vi "Lacie_20_Convertion.vi"(1 "Path":path) -> (0 "Path 2":path)   [LabVIEW 2010]
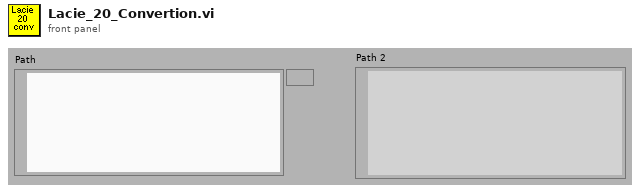
[diagram p1: front panel]
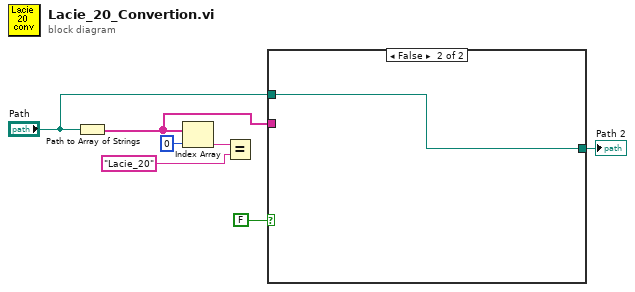
[diagram p0: block diagram]
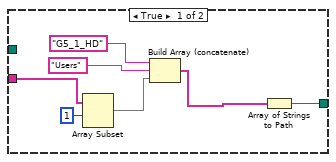
[diagram p2: hidden frame]
diagram:
  n1 = Path to Array of Strings(0:"Path") -> (2:w2:string[])  [unwired: 1 out]
  n2 = Index Array(array=w2, index=0) -> (element=w4:string)
  n3 = Equal?(x=w4, y="Lacie_20" ("regular expression")) -> ()  [unwired: 1 out]
  n4 = case shown="False" FALSE {
    tunnel: [w8 w15] -> w7
    tunnel: "Path" -> [_ w15]
    tunnel: w2 -> [w12 _]
    frame True {
      n5 = Array Subset(array=w12, index=1) -> (w10:string[])  [unwired: 1 in]
      n6 = Build Array (concatenate)("G5_1_HD", "Users", w10) -> (w9:string[])
      n7 = Array of Strings to Path(0:w9) -> (2:w8:path)  [unwired: 1 out]
    }
    frame False {
    }
  }
  "Path 2" <- w7
